vi "APC_SIL0_TraceHarness.vi"() -> ()   [LabVIEW 2020]
uses:
  <vilib>/Utility/file.llb/Read Delimited Spreadsheet (DBL).vi
  <vilib>/Utility/file.llb/Write Delimited Spreadsheet (DBL).vi
  <vilib>/Utility/file.llb/Write Delimited Spreadsheet (string).vi
panel:
  out "9049_CalculatedVariablesRaster":dbl[](array[numeric])
  out "SyncCylPres":dbl[][](graph)
  in  "Trace Folder":path
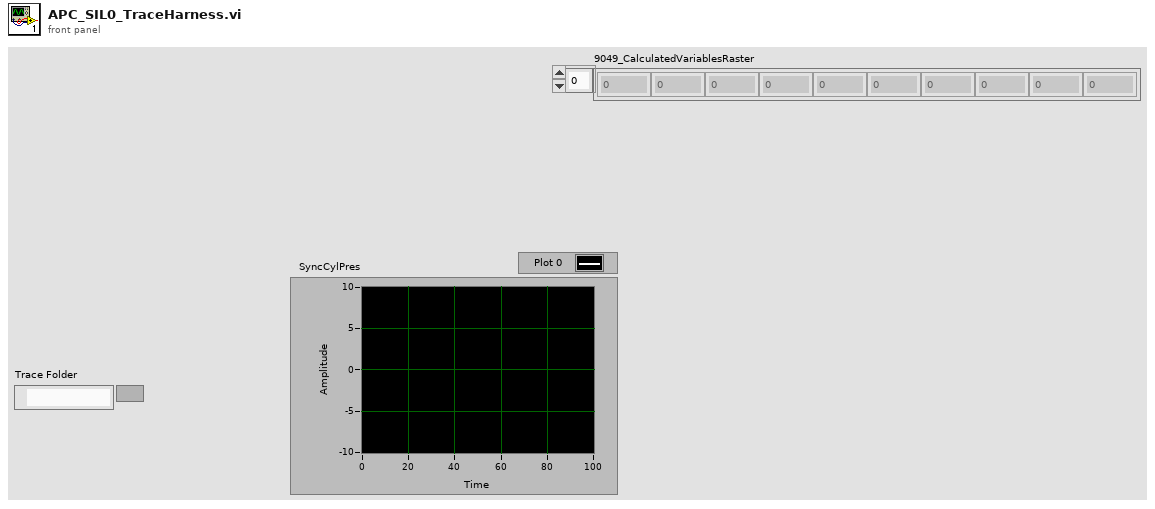
[diagram p1: front panel]
types:
  T1 = cluster{"IIR LowPass":cluster{"filter structure":enum32{"IIR 2nd Order", "IIR 4th Order"}, "Reverse Coefficients":dbl[], "Forward Coefficients":dbl[]}, "IIR HighPass":cluster{"filter structure":enum32{"IIR 2nd Order", "IIR 4th Order"}, "Reverse Coefficients":dbl[], "Forward Coefficients":dbl[]}}
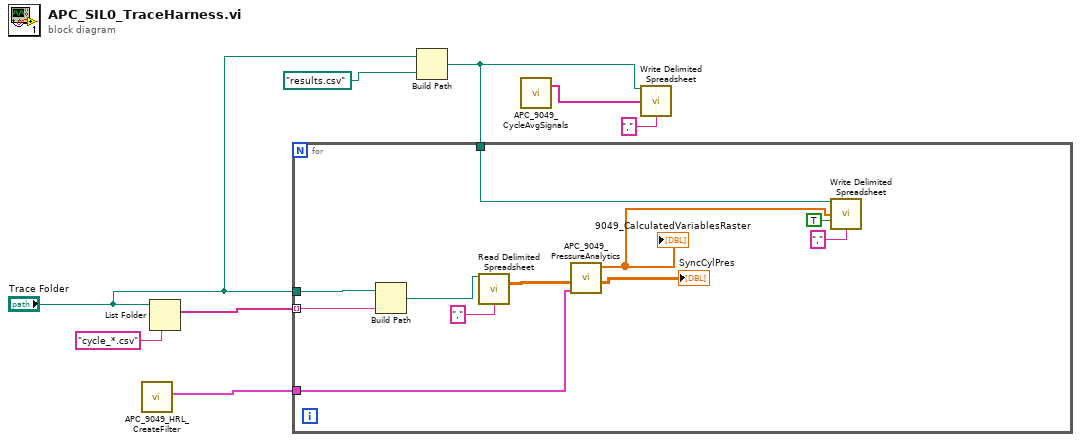
[diagram p0: block diagram]
diagram:
  n1 = call "APC_9049_HRL_CreateFilter.vi"() -> ("FilterCoefs"=w5:T1)  [unwired: 11 in]
  n2 = List Folder(path="Trace Folder", pattern="cycle_*.csv") -> (filenames=w6:string[])  [unwired: 2 in, 3 out]
  n3 = Build Path(base path="Trace Folder", name or relative path=path "results.csv") -> (appended path=w2:path)
  n4 = for {
    tunnel: w6 -> [w18] mode=indexing
    tunnel: "Trace Folder" -> [w19]
    tunnel: w5 -> [w14]
    tunnel: w2 -> [w10]
    n5 = Build Path(base path=w19, name or relative path=w18) -> (appended path=w17:path)
    n6 = call-poly <vilib>:"Read Delimited Spreadsheet.vi"("file path (dialog if empty)"=w17, "delimiter (\\t)"="," ("delimiter (\\t)")) -> ("all rows"=w15:dbl[][])  [unwired: 8 in, 5 out]
    n7 = call "APC_9049_PressureAnalytics.vi"("FilterCoefs"=w14, "AIdata [bar]"=w15) -> ("SyncCylPres [bar]"=→"SyncCylPres":dbl[][], "9049_CalculatedVariablesRaster"=w9:dbl[])  [unwired: 4 in]
    "9049_CalculatedVariablesRaster" <- w9
    n8 = call-poly <vilib>:"Write Delimited Spreadsheet.vi"("file path (dialog if empty)"=w10, "1D data"=w9, "append to file? (new file:F)"=TRUE, "delimiter (\\t)"="," ("delimiter (\\t)")) -> ()  [unwired: 10 in, 2 out]
  }
  n9 = call "APC_9049_CycleAvgSignals.vi"() -> ("CRIo9049_CycleAvgSignals"=w7:string[])  [unwired: 3 in]
  n10 = call-poly <vilib>:"Write Delimited Spreadsheet.vi"("file path (dialog if empty)"=w2, "1D data"=w7, "delimiter (\\t)"="," ("delimiter (\\t)")) -> ()  [unwired: 11 in, 2 out]
